vi "PruebaAutoR.vi"() -> ()   [LabVIEW 2014, in "MSX-E3711_dll.lvlib"]
uses:
  MSX-E3711_dll.lvlib
  Typedef/Config Data.ctl
  Typedef/Connection Data.ctl
  E:/Repositorio Magnis/INF002/v0/Modules/HAL/Drivers/Sync/ADDI-DATA MSX-E3711/API/MSXE371x.dll
  MSXE371x.dll
  E:/Repositorio Magnis/INF002/v0/Modules/HAL/Drivers/Sync/ADDI-DATA MSX-E3711/API/MXCommon.dll
  MXCommon.dll
  Typedef/Adquisition Data.ctl
  Typedef/Calibration Data.ctl
panel:
  out "Cluster Calibration":T1
  in  "Transductores":bool[][](array[boolean])
  out "error out":errorcluster
  in  "error in (no error)":errorcluster
  out "Adquisition Data":T2
  in  "stop":bool
  in  "Connection Data In":T3
  in  "Config Data":T4
  # "Information"
  # "HardwareTriggerEdge"
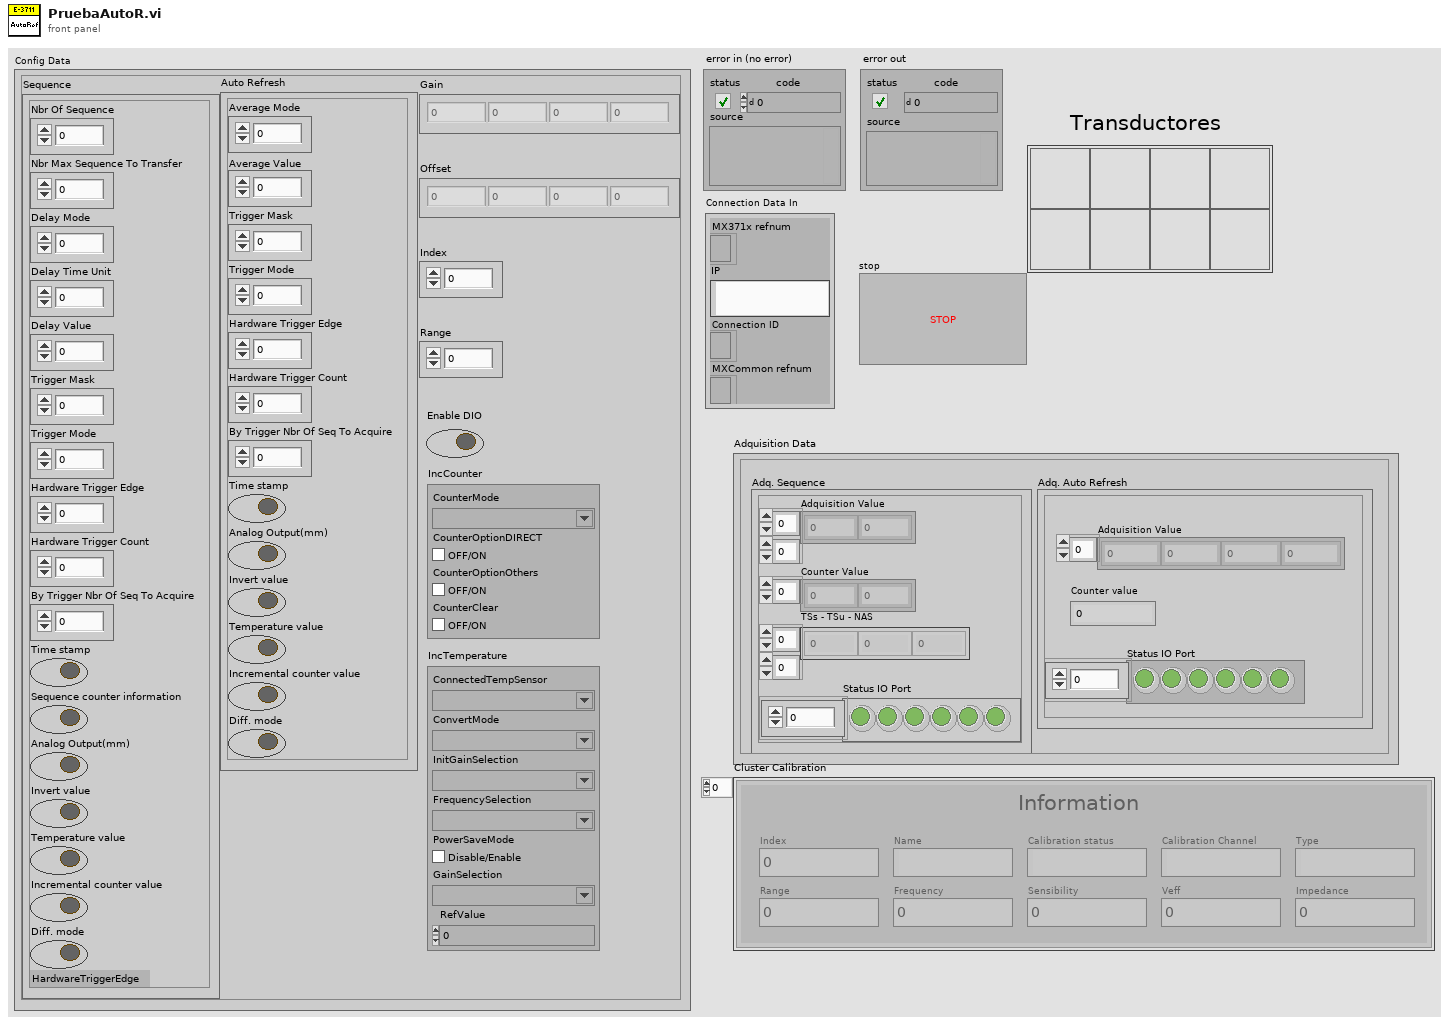
[diagram p1: front panel]
types:
  T1 = typedef "MSX-E3711_dll.lvlib/Calibration Data.ctl" = cluster{"Calibration status":string, "Name":string, "Index":u64, "Range":dbl, "Sensibility":dbl, "Veff":dbl, "Frequency":u64, "Impedance":u64, "Type":string, "Calibration Channel":string}[]
  T2 = typedef "MSX-E3711_dll.lvlib/Adquisition Data.ctl" = cluster{"Adq. Sequence":cluster{"Adquisition Value":u32[][], "Counter Value":u32[], "TSs - TSu - NAS":u64[][], "Status IO Port":bool[]}, "Adq. Auto Refresh":cluster{"Adquisition Value":u64[], "Status IO Port":bool[], "Counter value":u64}}
  T3 = typedef "MSX-E3711_dll.lvlib/Connection Data.ctl" = cluster{"MX371x refnum":refnum<k24>, "IP":string, "Connection ID ":refnum<k5>, "MXCommon refnum":refnum<k24>}
  T4 = typedef "MSX-E3711_dll.lvlib/Config Data.ctl" = cluster{"Auto Refresh":cluster{"Average Mode":u64, "Average Value":u64, "Trigger Mask":u64, "Trigger Mode":u64, "Hardware Trigger Edge":u64, "Hardware Trigger Count":u64, "By Trigger Nbr Of Seq To Acquire":u64, "Time stamp":bool, "Analog Output(mm)":bool, "Invert value":bool, "Temperature value":bool, "Incremental counter value":bool, "Diff. mode":bool}, "Gain":sgl[], "Offset":sgl[], "Index":u64, "Range":sgl, "Sequence":cluster{"Nbr Of Sequence":u64, "Nbr Max Sequence To Transfer":u64, "Delay Mode":u64, "Delay Time Unit":u64, "Delay Value":u64, "Trigger Mask":u64, "Trigger Mode":u64, "Hardware Trigger Edge":u64, "Hardware Trigger Count":u64, "By Trigger Nbr Of Seq To Acquire":u64, "Time stamp":bool, "Sequence counter information":bool, "Analog Output(mm)":bool, "Invert value":bool, "Temperature value":bool, "Incremental counter value":bool, "Diff. mode":bool}, "Enable DIO":bool, "IncCounter":cluster{"CounterMode":string, "CounterOptionDIRECT  ":bool, "CounterOptionOthers":bool, "CounterClear ":bool}, "IncTemperature":cluster{"ConnectedTempSensor":string, "ConvertMode":string, "InitGainSelection":string, "FrequencySelection":string, "PowerSaveMode":bool, "GainSelection":string, "RefValue":dbl}}
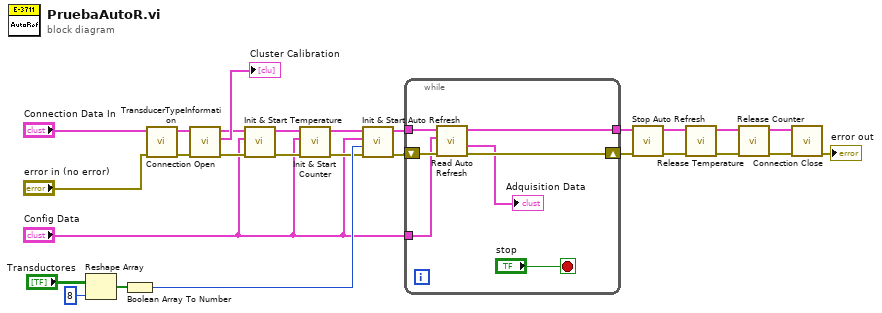
[diagram p0: block diagram]
diagram:
  n1 = Reshape Array("Transductores", 8 ("dimension size")) -> (w20:bool[])
  n2 = Boolean Array To Number(Boolean array=w20) -> (number=w17:u64)
  n3 = call "Connection Open.vi"("error in (no error)"="error in (no error)", "Connection Data In"="Connection Data In") -> ("error out"=w15:errorcluster, "Connection Data Out"=w16:T3)  [unwired: 8 in]
  n4 = call "TransducerTypeInformation.vi"("error in (no error)"=w15, "Connection Data In"=w16) -> ("error out"=w10:errorcluster, "Cluster Calibration"=→"Cluster Calibration":T1, "Connection Data Out"=w13:T3)  [unwired: 7 in]
  n5 = call "Init & Start Temperature.vi"("error in (no error)"=w10, "Config Data"="Config Data", "Connection Data In"=w13) -> ("error out"=w9:errorcluster, "Connection Data Out"=w12:T3)  [unwired: 7 in]
  n6 = call "Init & Start Counter.vi"("error in (no error)"=w9, "Config Data"="Config Data", "Connection Data In"=w12) -> ("error out"=w8:errorcluster, "Connection Data Out"=w11:T3)  [unwired: 7 in]
  n7 = call "Init & Start Auto Refresh.vi"("error in (no error)"=w8, "Channel Mask"=w17, "Config Data"="Config Data", "Connection Data In"=w11) -> ("error out"=w23:errorcluster, "Connection Data Out"=w24:T3)  [unwired: 6 in]
  n8 = while {
    shift-right: [w33] -> w25
    shift-left: w23 -> [w30]
    tunnel: w24 -> [w31]
    tunnel: [w32] -> w26
    tunnel: "Config Data" -> [w28]
    stop <- "stop" stop-if-true
    n9 = call "Read Auto Refresh.vi"("error in (no error)"=w30, "Config Data"=w28, "Connection Data In"=w31) -> ("error out"=w33:errorcluster, "Adquisition Data Out"=→"Adquisition Data":T2, "Connection Data Out"=w32:T3)  [unwired: 6 in]
  }
  n10 = call "Stop Auto Refresh.vi"("error in (no error)"=w25, "Connection Data In"=w26) -> ("error out"=w2:errorcluster, "Connection Data Out"=w7:T3)  [unwired: 8 in]
  n11 = call "Release Temperature.vi"("error in (no error)"=w2, "Connection Data In"=w7) -> ("error out"=w3:errorcluster, "Connection Data Out"=w6:T3)  [unwired: 8 in]
  n12 = call "Release Counter.vi"("error in (no error)"=w3, "Connection Data In"=w6) -> ("error out"=w4:errorcluster, "Connection Data Out"=w5:T3)  [unwired: 8 in]
  n13 = call "Connection Close.vi"("error in (no error)"=w4, "Connection Data In"=w5) -> ("error out"=→"error out":errorcluster)  [unwired: 8 in, 1 out]
